vi "Oxford1820 Client.vi"(8 "error in (no error)":errorcluster, 9 "Data":variant, 10 "Commands":T1, 11 "Instrument.1820 in":refnum<class "Instrument.Oxford1820.lvclass">) -> (0 "error out":errorcluster, 1 "Data out":variant, 3 "Instrument.1820 out":refnum<class "Instrument.Oxford1820.lvclass">)   [LabVIEW 2016, in "Instrument.Oxford1820.lvclass"]
uses:
  Instrument.Oxford1820.lvclass
  Typedefs/Instrument.Oxford1820.Commands-enum.ctl
  <userlib>/LevyLab/Levylab Instruments/SMOs/RemoteControl.STM/RemoteControl.STM.lvclass
  C:/Program Files (x86)/National Instruments/LabVIEW 2016/user.lib/LevyLab/Levylab Instruments/SMOs/RemoteControl/RemoteControl.lvclass
  <userlib>/LevyLab/Levylab Instruments/SMOs/RemoteControl/RemoteControl.lvclass
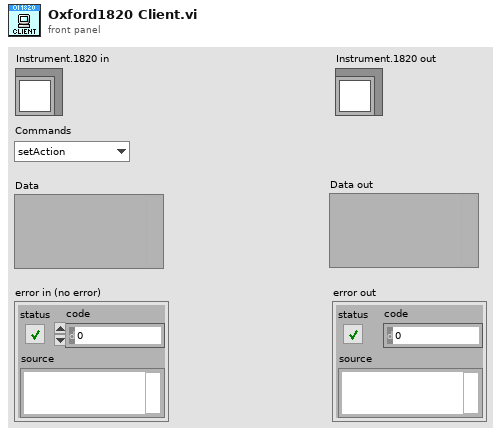
[diagram p1: front panel]
types:
  T1 = typedef "Instrument.Oxford1820.lvclass/Instrument.Oxford1820.Commands-enum.ctl" = enum16{"setAction", "setTarget", "setSwitchHeat", "setLambda", "setFillMode", "setNeedleValve", "setMagnetField", "getStatus", "getTarget", "getSwitchHeat", "getPSUField", "getMagnetField"}
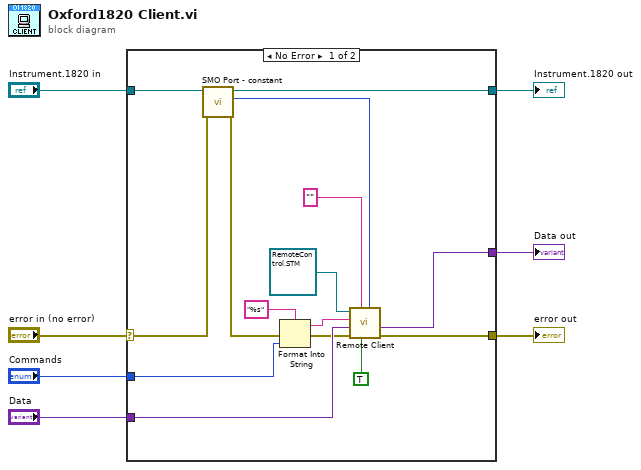
[diagram p0: block diagram]
diagram:
  n1 = case shown="No Error" "error in (no error)" {
    selector: "error in (no error)" -> [w10 w24]
    tunnel: "Data" -> [w22 _]
    tunnel: [w21 w24] -> w6
    tunnel: [w20 _] -> w5
    tunnel: "Commands" -> [w19 _]
    tunnel: "Instrument.1820 in" -> [w12 w23]
    tunnel: [w11 w23] -> w1
    frame No Error {
      n2 = call-dynamic "SMO Port - constant.vi"("error in (no error)"=w10, "Instrument.Oxford1820 in"=w12) -> ("error out"=w9:errorcluster, "Port"=w13:u16, "Instrument.Oxford1820 out"=w11:refnum<class "Instrument.Oxford1820.lvclass">)  [unwired: 7 in]
      n3 = Format Into String(format string="%s", error in=w9, w19) -> (resulting string=w17:string, error out=w16:errorcluster)  [unwired: 1 in]
      n4 = call <userlib>:"Remote Client.vi"("Port"=w13, "Wait for Response?"=TRUE, "address"="", "error in (no error)"=w16, "Data"=w22, "Command"=w17, "RemoteControl in"=refnum<class "RemoteControl.STM.lvclass"> refnum ("RemoteControl.STM in")) -> ("error out"=w21:errorcluster, "Data out"=w20:variant)  [unwired: 1 in, 2 out]
    }
    frame Error {
    }
  }
  "Instrument.1820 out" <- w1
  "error out" <- w6
  "Data out" <- w5
